vi "Modify BFIC in phase table.vi"() -> ()   [LabVIEW 2023, in "HAPS.lvlib"]
uses:
  HAPS.lvlib
  <vilib>/Utility/file.llb/Read Delimited Spreadsheet (string).vi
  HAPS_MCU_ELE_Func.ctl
  R_S/R_S.lvlib
  HAPS_SerialPort.ctl
panel:
  in  "Phase Offset?":i32
  in  "chain ID?":i32
  in  "chain ID?":i32
  in  "group?":i32
  in  "array id?":i32
  in  "file path":path=path "D:/_Project/_Code/LabVIEW/_CLC_Gen4/CLC_LV2023/CLC_Cali/Log/HAPS/Preset.csv"
  out "status":bool
  out "ele phase":i32
  out "ele gain":i32
  out "channel":i32
  out "chain ID":i32
  out "group":i32
  out "array id":i32
  # "HAPS 24x24 Setting Manual In-Phase : \n                                                           Any BFIC"
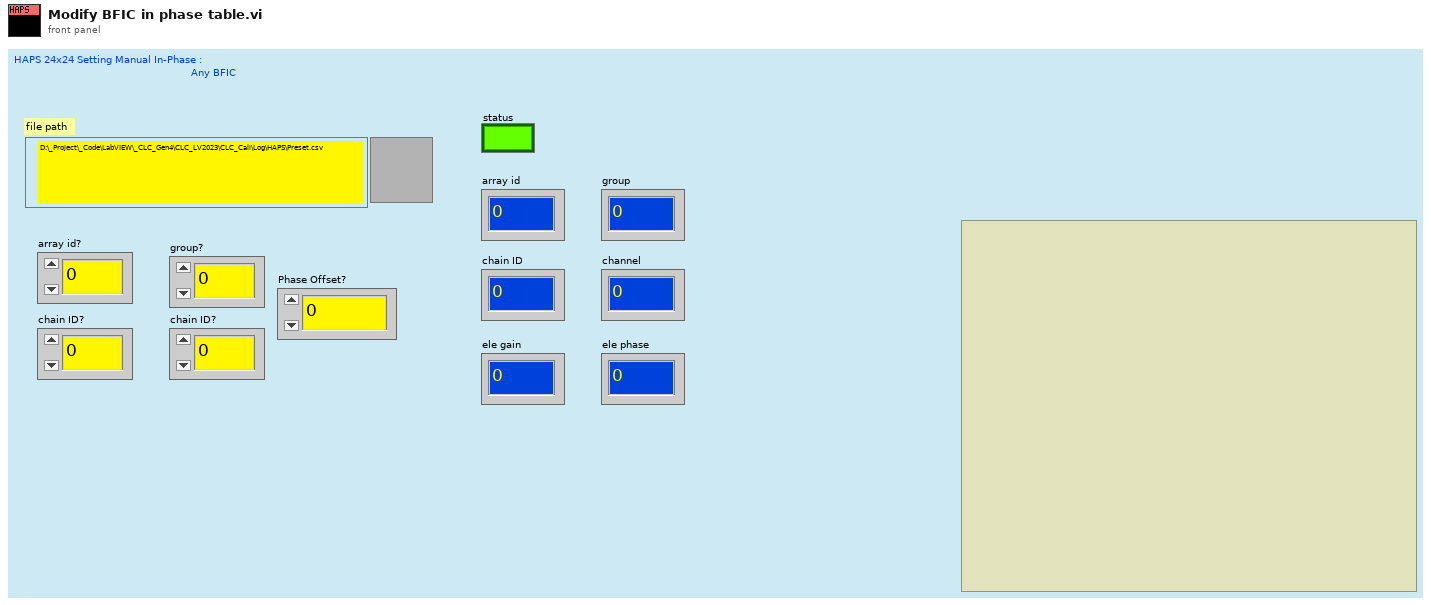
[diagram p1: front panel]
types:
  T1 = typedef "HAPS.lvlib/HAPS_SerialPort.ctl" = enum16{"Init", "Close", "CMD", "Flush"}
  T2 = typedef "HAPS.lvlib/HAPS_MCU_ELE_Func.ctl" = enum16{"array_init", "set_com_gain", "set_ch_gain_phase", "set_pd_range", "get_preamp_temp", "get_bfic_temp", "get_tx_pd", "ch_on", "ch_on_2", "ch_ctrl_all", "array_ctrl_src"}
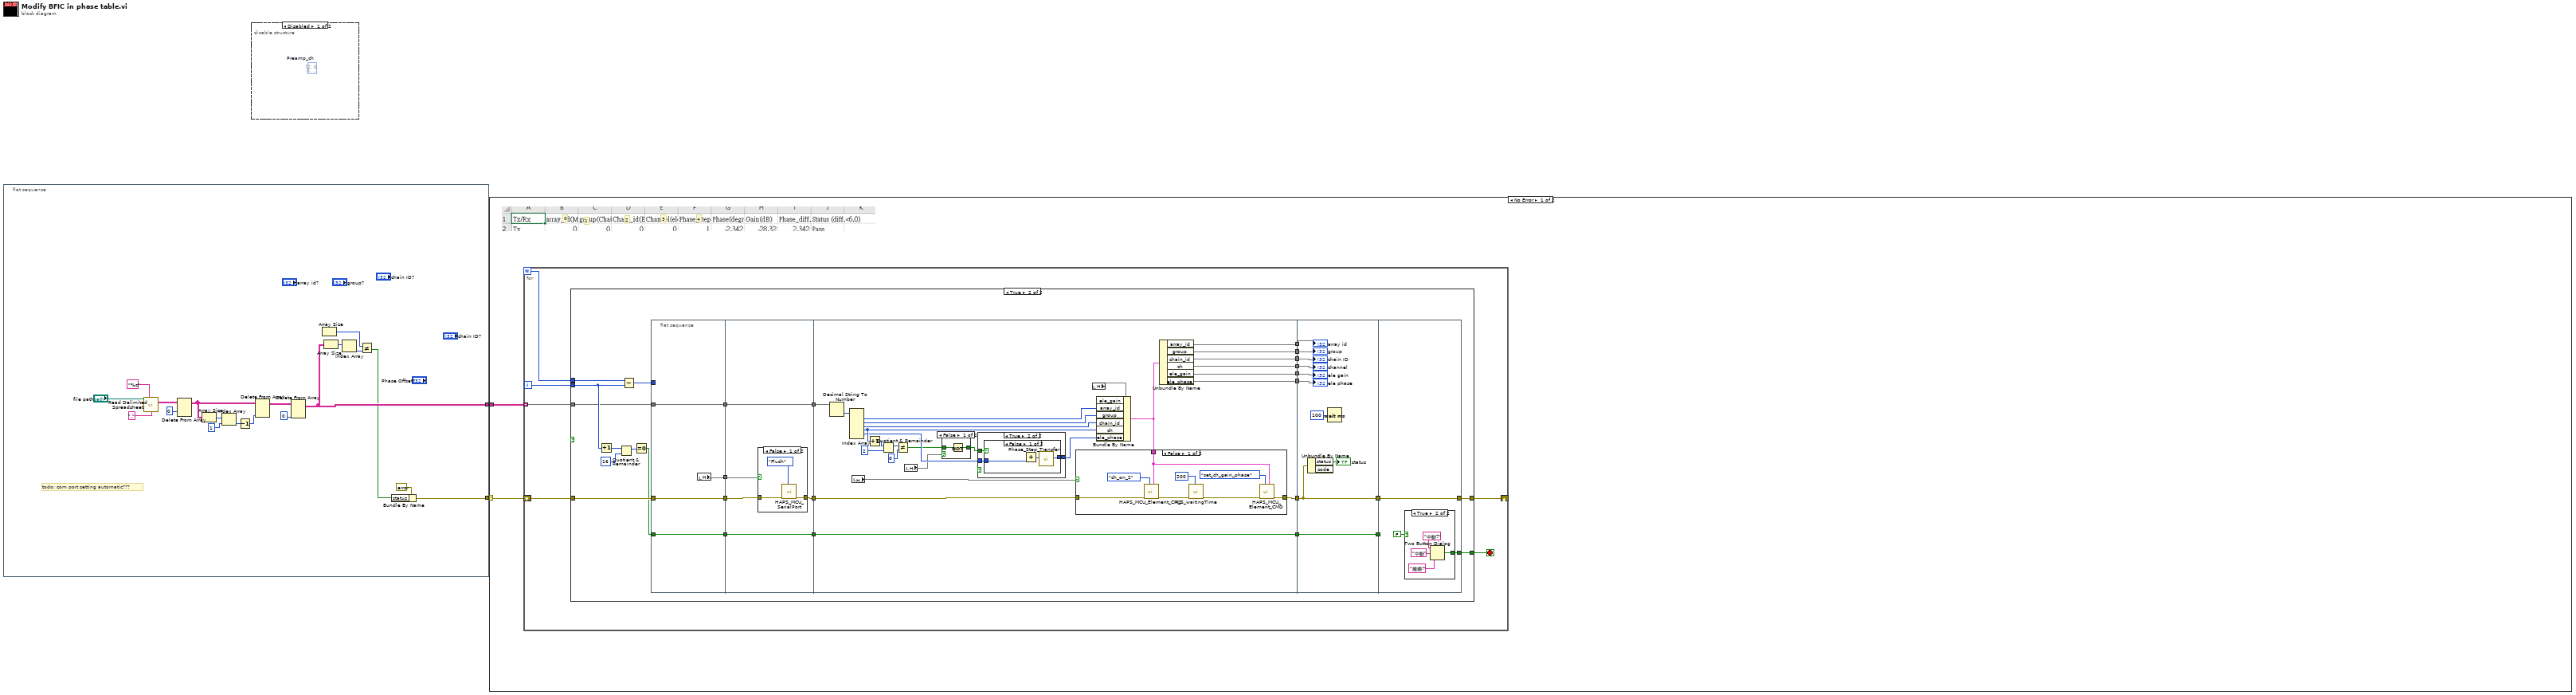
[diagram p0: block diagram]
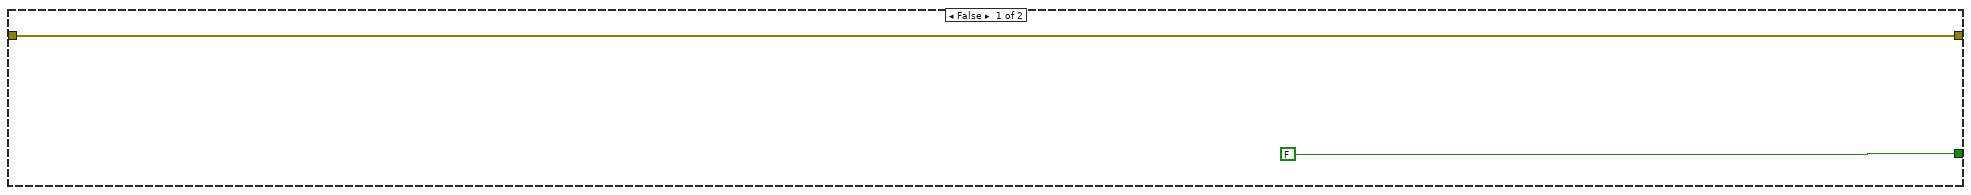
[diagram p3: hidden frame]
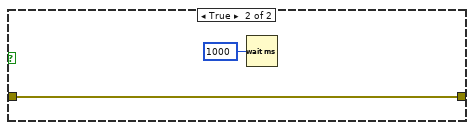
[diagram p8: hidden frame]
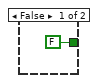
[diagram p9: hidden frame]
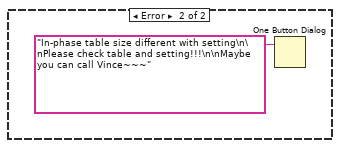
[diagram p10: hidden frame]
diagram:
  n1 = flat-sequence {
    tunnel: [w3] -> w2
    tunnel: [w9] -> w1
    frame #0 {
      # "todo: com port setting automatic???"
      n2 = call-poly <vilib>:"Read Delimited Spreadsheet.vi"("file path (dialog if empty)"="file path", "format (%s)"="%s" ("format (%.3f)"), "delimiter (\\t)"="," ("delimiter (\\t)")) -> ("all rows"=w19:string[][])  [unwired: 7 in, 5 out]
      n3 = Delete From Array(array=w19, index (row)=0) -> (array with subset deleted=w11:string[][])  [unwired: 2 in, 1 out]
      n4 = Array Size(array=w11) -> (size(s)=w17:i32[])
      n5 = Index Array(array=w17, index=1) -> (element=w14:i32)
      n6 = Decrement(x=w14) -> (x-1=w16:i32)
      n7 = Delete From Array(array=w11, index (col)=w16) -> (array with subset deleted=w13:string[][])  [unwired: 2 in, 1 out]
      n8 = Delete From Array(array=w13, index (col)=0 ("index (row)")) -> (array with subset deleted=w9:string[][])  [unwired: 2 in, 1 out]
      n9 = Array Size() -> (size(s)=w7:i32)  [unwired: 1 in]
      n10 = Array Size(array=w9) -> (size(s)=w8:i32[])
      n11 = Index Array(array=w8) -> (element=w6:i32)  [unwired: 1 in]
      n12 = Not Equal?(x=w7, y=w6) -> (x != y?=w4:bool)
      n13 = Bundle By Name(cluster=errorcluster {"status"=FALSE, "code"=0, "source"=""} ("error out"), "status"=w4) -> (w3:errorcluster)
    }
  }
  n14 = disable-structure shown="Disabled" {
    frame Disabled {
      (unwired) i32[][] [[2, 0, 0, 8, 8, 10, 11, 9, 9, 1, 1, 3], [3, 1, 1, 9, 9, 11, 13, 15, 15, 7, 7, 5], [5, 7, 7, 15, 15, 13, 14, 14, 6, 6, 4, 12]]  # Preamp_ch
    }
    frame Enabled {
    }
  }
  n15 = case shown="No Error" w2 {
    selector: w2 -> [w22 _]
    tunnel: w1 -> [w23 _]
    frame No Error {
      # "4"
      # "3"
      # "2"
      # "1"
      # "0"
      n16 = for {
        N -> [w28]
        tunnel: w23 -> [w26] mode=indexing
        shift-right: [w30] -> w24
        shift-left: w22 -> [w29]
        i -> [w27]
        stop <- w25 stop-if-true
        n17 = case shown="True" {
          selector: _ -> [_ _]
          tunnel: [w31 w44] -> w30
          tunnel: w29 -> [w31 w43]
          tunnel: w28 -> [_ w42]
          tunnel: w27 -> [_ w41]
          tunnel: w26 -> [_ w40]
          tunnel: [FALSE ("T button?") w34] -> w25
          frame False {
          }
          frame True {
            n18 = Increment(x=w41) -> (x+1=w38:i32)
            n19 = Quotient & Remainder(x=w38, y=16) -> (x-y*floor(x/y)=w36:i32)  [unwired: 1 out]
            n20 = Subtract(x=w42, y=w41) -> (x-y=w39:i32)
            n21 = Equal To 0?(x=w36) -> (x = 0?=w35:bool)
            n22 = flat-sequence {
              tunnel: w39 -> [_]
              tunnel: w43 -> [w63]
              tunnel: w40 -> [w64]
              tunnel: [w64] -> w60
              tunnel: [w63] -> w59
              tunnel: w35 -> [w62]
              tunnel: [w62] -> w58
              tunnel: [w61] -> w33
              tunnel: [w69] -> w57
              tunnel: [w68] -> w56
              tunnel: w60 -> [w69]
              tunnel: w59 -> [w67]
              tunnel: w58 -> [w66]
              tunnel: [w66] -> w55
              tunnel: w33 -> [w65]
              tunnel: w57 -> [w101]
              tunnel: w56 -> [w99]
              tunnel: [w87] -> w54
              tunnel: [w97] -> w53
              tunnel: [w96] -> w52
              tunnel: [w95] -> w51
              tunnel: [w94] -> w50
              tunnel: [w93] -> w49
              tunnel: [w92] -> w48
              tunnel: w55 -> [w88]
              tunnel: [w88] -> w47
              tunnel: w54 -> [w125]
              tunnel: w53 -> [w133]
              tunnel: w52 -> [w132]
              tunnel: w51 -> [w131]
              tunnel: w50 -> [w130]
              tunnel: w49 -> [w129]
              tunnel: w48 -> [w128]
              tunnel: [w125] -> w46
              tunnel: w47 -> [w126]
              tunnel: [w126] -> w45
              tunnel: w46 -> [w136]
              tunnel: w45 -> [_]
              tunnel: [w136] -> w44
              tunnel: [w135] -> w34
              frame #0 {
                n23 = local read item#-1() -> (w61)
              }
              frame #1 {
                n24 = case shown="False" w65 {
                  tunnel: [w72 w73] -> w68
                  tunnel: w67 -> [w71 w73]
                  frame False {
                    n25 = call "HAPS_MCU_SerialPort.vi"("HAPS_SerialPort_Func"=HAPS_SerialPort."Flush", "error in"=w71) -> ("error out"=w72:errorcluster)  [unwired: 7 in, 2 out]
                  }
                  frame True {
                  }
                }
              }
              frame #2 {
                n26 = Decimal String To Number(string=w101) -> (number=w100:i32[])  [unwired: 2 in, 1 out]
                n27 = Index Array(array=w100) -> (element #1=w98:i32, element #2=w91:i32, element #3=w90:i32, element #4=w84:i32, element #5=w80:i32)  [unwired: 6 in, 1 out]
                n28 = local read item#-1() -> (w86)
                n29 = Increment(x=w84) -> (x+1=w77:i32)
                n30 = Quotient & Remainder(x=w77, y=2) -> (x-y*floor(x/y)=w82:i32)  [unwired: 1 out]
                n31 = Not Equal?(x=w82, y=0) -> (x != y?=w75:bool)
                n32 = local read item#-1() -> (w76)
                n33 = case shown="False" w76 {
                  tunnel: w75 -> [w103 w104]
                  tunnel: [w102 w104] -> w74
                  frame False {
                    n34 = Not(x=w103) -> (.not. x?=w102:bool)
                  }
                  frame True {
                  }
                }
                n35 = case shown="True" w78 {
                  tunnel: w80 -> [w105 w108]
                  tunnel: w74 -> [_ w107]
                  tunnel: [w105 w106] -> w79
                  frame False {
                  }
                  frame True {
                    n36 = case shown="False" w107 {
                      tunnel: w108 -> [w111 w112]
                      tunnel: [w109 w112] -> w106
                      frame False {
                        n37 = Add(y=w111) -> (x+y=w110:i32)  [unwired: 1 in]
                        n38 = call "Phase_Step_Transfer.vi"("Input_Phase_Step"=w110) -> ("Output_Phase_Step"=w109:i32)  [unwired: 10 in]
                      }
                      frame True {
                      }
                    }
                  }
                }
                n39 = local read item#-1() -> (w89)
                n40 = Bundle By Name(cluster=w89, "array_id"=w98, "group"=w91, "chain_id"=w90, "ch"=w84, "ele_phase"=w79) -> (w85:cluster{})  [unwired: 1 in]
                n41 = case shown="False" w86 {
                  tunnel: w99 -> [w120 w122]
                  tunnel: w85 -> [w119 _]
                  tunnel: [w118 w122] -> w87
                  frame False {
                    n42 = call "HAPS_MCU_Element_CMD.vi"("set_ele"=w119, "HAPS_MCU_ELE_Func."=HAPS_MCU_ELE_Func."ch_on_2", "error in"=w120) -> ("error out"=w114:errorcluster)  [unwired: 7 in, 1 out]
                    n43 = call "R_S_waitingTime.vi"("Waiting Time(ms)"=u32 200, "error in"=w114) -> ("error out"=w113:errorcluster)  [unwired: 9 in]
                    n44 = call "HAPS_MCU_Element_CMD.vi"("set_ele"=w119, "HAPS_MCU_ELE_Func."=HAPS_MCU_ELE_Func."set_ch_gain_phase", "error in"=w113) -> ("error out"=w118:errorcluster)  [unwired: 7 in, 1 out]
                  }
                  frame True {
                    n45 = Wait (ms)(milliseconds to wait=u32 1000) -> ()  [unwired: 1 out]
                  }
                }
                n46 = Unbundle By Name(w85) -> ("array_id"=w97, "group"=w96, "chain_id"=w95, "ch"=w94, "ele_gain"=w93, "ele_phase"=w92)
              }
              frame #3 {
                n47 = Unbundle By Name(w125) -> ("status"=→"status":bool, "code"=w123:i32)
                n48 = Wait (ms)(milliseconds to wait=u32 100) -> ()  [unwired: 1 out]
                "group" <- w132
                "chain ID" <- w131
                "channel" <- w130
                "ele gain" <- w129
                "ele phase" <- w128
                "array id" <- w133
              }
              frame #4 {
                n49 = case shown="True" FALSE {
                  tunnel: [FALSE ("T button?") w140] -> w135
                  frame False {
                  }
                  frame True {
                    n50 = Two Button Dialog(message="中斷?", 1:"繼續!" ("F button name (\"Cancel\")"), 2:"中斷" ("T button name (\"OK\")")) -> (T button?=w140:bool)
                  }
                }
              }
            }
          }
        }
      }
    }
    frame Error {
      n51 = One Button Dialog(message="In-phase table size different with setting\n\nPlease check table and setting!!!\n\nMaybe you can call Vince~~~") -> ()  [unwired: 1 in, 1 out]
    }
  }
